vi "Panel Resized.vi"(8 "error in (no error)":errorcluster, 11 "UI_Top in":refnum<class "UI_Top.lvclass">) -> (0 "error out":errorcluster, 3 "UI_Top out":refnum<class "UI_Top.lvclass">)   [LabVIEW 2021, in "UI_Top.lvclass"]
uses:
  UI_Top.lvclass
  C:/Program Files (x86)/National Instruments/LabVIEW 2021/user.lib/John_Lib/AbstractActorTemplate/AbstractActorTemplate/UIActorTop.lvclass
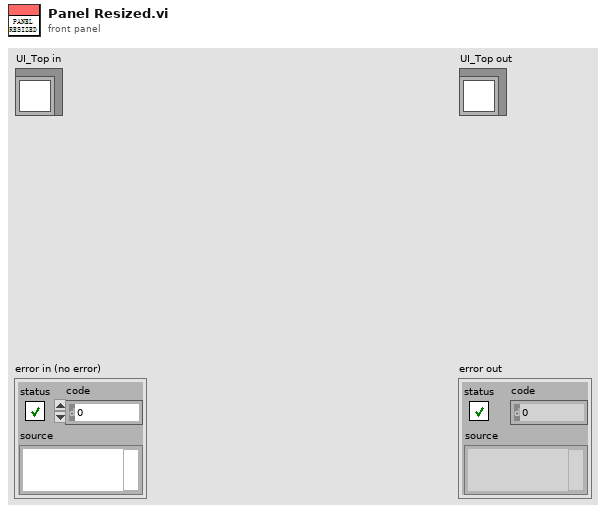
[diagram p1: front panel]
types:
  T1 = typedef "LVRectTypeDef.ctl" = cluster{"Left":i16, "Top":i16, "Right":i16, "Bottom":i16}
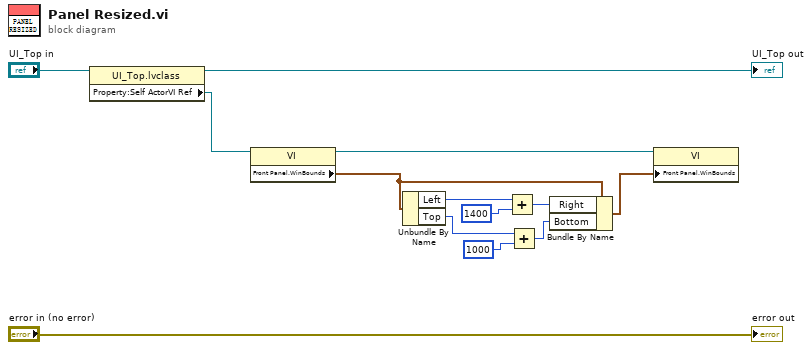
[diagram p0: block diagram]
diagram:
  n1 = property class="UI_Top.lvclass"(reference="UI_Top in") -> (reference out=→"UI_Top out":refnum<class "UI_Top.lvclass">, "Property:Self ActorVI Ref"=w12:refnum<vi>)  [unwired: 1 in, 1 out]
  n2 = property class="VI"(reference=w12) -> (reference out=w2:refnum<vi>, "Front Panel.WinBounds"=w3:T1)  [unwired: 1 in, 1 out]
  n3 = Unbundle By Name(w3) -> ("Left"=w4:i16, "Top"=w6:i16)
  n4 = Add(x=w4, y=i16 1400 ("y 2")) -> (x+y=w5:i16)
  n5 = Add(x=w6, y=i16 1000) -> (x+y=w7:i16)
  n6 = Bundle By Name(cluster=w3, "Right"=w5, "Bottom"=w7) -> (w1:T1)
  n7 = property class="VI"(reference=w2, "Front Panel.WinBounds"=w1) -> ()  [unwired: 1 in, 2 out]
  "error out" <- "error in (no error)"
